vi "stepper.vi"() -> ()   [LabVIEW 2016]
panel:
  in  "Counter clockwise rotation":bool
  in  "Clockwise rotation":bool
  out "Gauge":dbl(knob) scale=0.0..4.0
  out "D":bool
  out "C":bool
  out "B":bool
  out "A":bool
  # "When set closes the gripper"
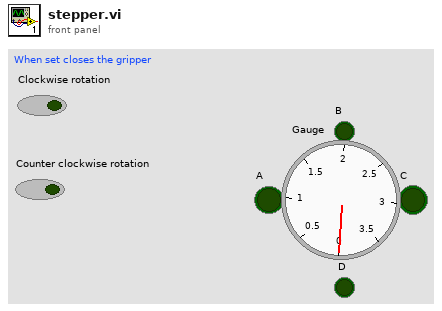
[diagram p1: front panel]
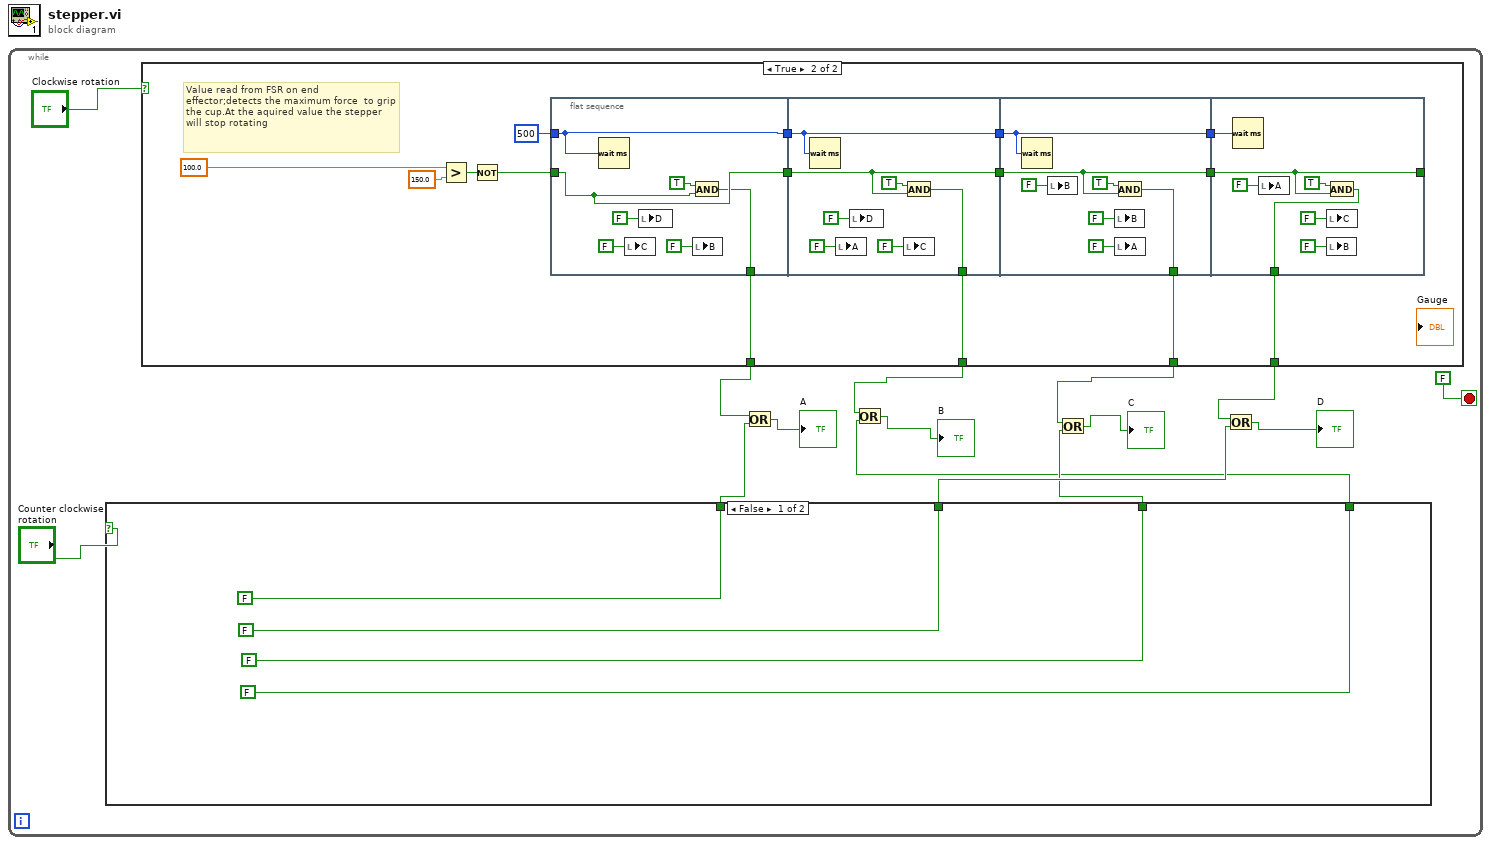
[diagram p0: block diagram]
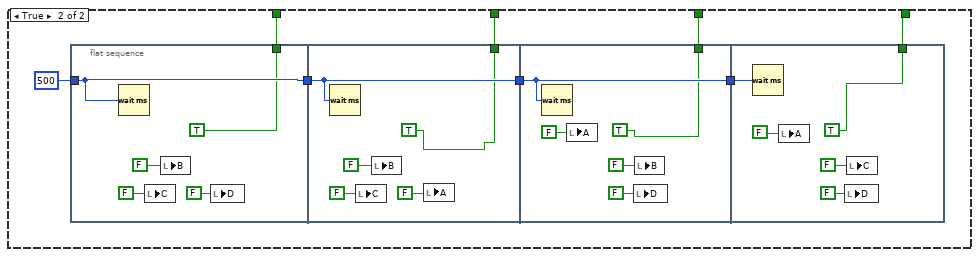
[diagram p2: hidden frame]
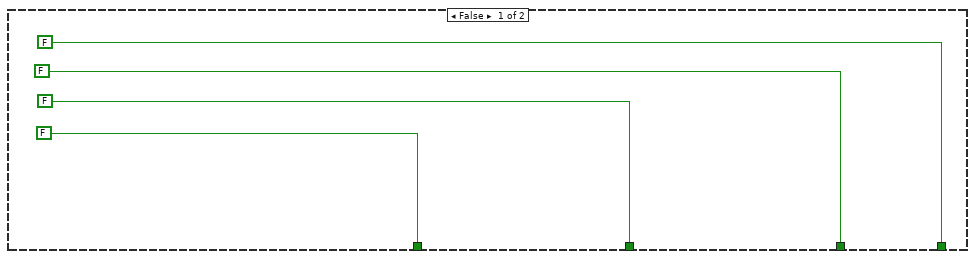
[diagram p3: hidden frame]
diagram:
  n1 = while {
    stop <- FALSE stop-if-true
    n2 = case shown="False" "Counter clockwise rotation" {
      tunnel: [FALSE w23] -> w4
      tunnel: [FALSE w22] -> w3
      tunnel: [FALSE w21] -> w2
      tunnel: [FALSE w20] -> w1
      frame False {
      }
      frame True {
        n3 = flat-sequence {
          tunnel: 500 -> [w32]
          tunnel: [w32] -> w27
          tunnel: [TRUE] -> w23
          tunnel: w27 -> [w37]
          tunnel: [w37] -> w26
          tunnel: [TRUE] -> w22
          tunnel: w26 -> [w42]
          tunnel: [w42] -> w25
          tunnel: [TRUE] -> w21
          tunnel: w25 -> [w47]
          tunnel: [TRUE] -> w20
          frame #0 {
            n4 = Wait (ms)(milliseconds to wait=w32) -> ()  [unwired: 1 out]
            n5 = local write "C"(FALSE) -> ()
            n6 = local write "B"(FALSE) -> ()
            n7 = local write "D"(FALSE) -> ()
          }
          frame #1 {
            n8 = Wait (ms)(milliseconds to wait=w37) -> ()  [unwired: 1 out]
            n9 = local write "C"(FALSE) -> ()
            n10 = local write "B"(FALSE) -> ()
            n11 = local write "A"(FALSE) -> ()
          }
          frame #2 {
            n12 = Wait (ms)(milliseconds to wait=w42) -> ()  [unwired: 1 out]
            n13 = local write "A"(FALSE) -> ()
            n14 = local write "D"(FALSE) -> ()
            n15 = local write "B"(FALSE) -> ()
          }
          frame #3 {
            n16 = Wait (ms)(milliseconds to wait=w47) -> ()  [unwired: 1 out]
            n17 = local write "A"(FALSE) -> ()
            n18 = local write "D"(FALSE) -> ()
            n19 = local write "C"(FALSE) -> ()
          }
        }
      }
    }
    n20 = case shown="True" "Clockwise rotation" {
      tunnel: [FALSE w55] -> w11
      tunnel: [FALSE w54] -> w6
      tunnel: [FALSE w53] -> w7
      tunnel: [FALSE w52] -> w10
      frame False {
      }
      frame True {
        # "Value read from FSR on end effector;detects the maximum force  to grip the cup.At the aquired value the stepper will stop rotating"
        n21 = Greater?(x=100.0, y=150.0) -> (0:w58:bool)
        n22 = Not(x=w58) -> (.not. x?=w60:bool)
        n23 = flat-sequence {
          tunnel: 500 -> [w68]
          tunnel: w60 -> [w69]
          tunnel: [w69] -> w66
          tunnel: [w68] -> w65
          tunnel: [w67] -> w55
          tunnel: w66 -> [w76]
          tunnel: [w76] -> w64
          tunnel: w65 -> [w75]
          tunnel: [w75] -> w63
          tunnel: [w74] -> w54
          tunnel: w64 -> [w83]
          tunnel: [w83] -> w62
          tunnel: w63 -> [w82]
          tunnel: [w82] -> w61
          tunnel: [w81] -> w53
          tunnel: w62 -> [w89]
          tunnel: w61 -> [w90]
          tunnel: [w89] -> _
          tunnel: [w88] -> w52
          frame #0 {
            n24 = Wait (ms)(milliseconds to wait=w68) -> ()  [unwired: 1 out]
            n25 = local write "C"(FALSE) -> ()
            n26 = local write "D"(FALSE) -> ()
            n27 = And(x=TRUE, y=w69) -> (x .and. y?=w67:bool)
            n28 = local write "B"(FALSE) -> ()
          }
          frame #1 {
            n29 = Wait (ms)(milliseconds to wait=w75) -> ()  [unwired: 1 out]
            n30 = local write "A"(FALSE) -> ()
            n31 = local write "D"(FALSE) -> ()
            n32 = And(x=TRUE, y=w76) -> (x .and. y?=w74:bool)
            n33 = local write "C"(FALSE) -> ()
          }
          frame #2 {
            n34 = Wait (ms)(milliseconds to wait=w82) -> ()  [unwired: 1 out]
            n35 = local write "B"(FALSE) -> ()
            n36 = And(x=TRUE, y=w83) -> (x .and. y?=w81:bool)
            n37 = local write "B"(FALSE) -> ()
            n38 = local write "A"(FALSE) -> ()
          }
          frame #3 {
            n39 = Wait (ms)(milliseconds to wait=w90) -> ()  [unwired: 1 out]
            n40 = local write "A"(FALSE) -> ()
            n41 = And(x=TRUE, y=w89) -> (x .and. y?=w88:bool)
            n42 = local write "C"(FALSE) -> ()
            n43 = local write "B"(FALSE) -> ()
          }
        }
      }
    }
    n44 = Or(x=w11, y=w4) -> (x .or. y?=→"A":bool)
    n45 = Or(x=w6, y=w1) -> (x .or. y?=→"B":bool)
    n46 = Or(x=w7, y=w2) -> (x .or. y?=→"C":bool)
    n47 = Or(x=w10, y=w3) -> (x .or. y?=→"D":bool)
  }
